vi "Read TSP Link Synchronization Line Data.vi"(8 "error in (no error)":errorcluster, 9 "TSP Link Line (1)":i32=1, 10 "Data Type (0: Bit)":i32(ring) items=["Bit", "Port"], 11 "VISA resource name":refnum<visa-resource-name>) -> (0 "error out":errorcluster, 1 "Port":i32, 2 "Bit":i32, 3 "VISA resource name out":refnum<visa-resource-name>)   [LabVIEW 2017, in "Keithley 2600 Series.lvlib"]
doc: "Returns the TSP-Link synchronization line data.\n\n<b>Note:</b>\nThis VI is not available on models 2604B, 2614B, 2634B."
uses:
  <instrlib>/Keithley 2600 Series/Keithley 2600 Series.lvlib
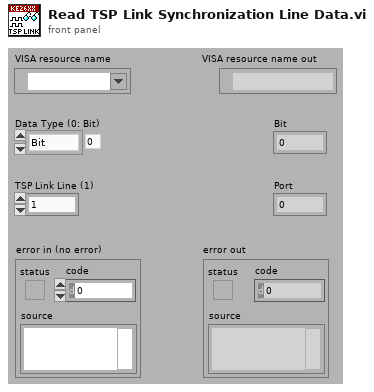
[diagram p1: front panel]
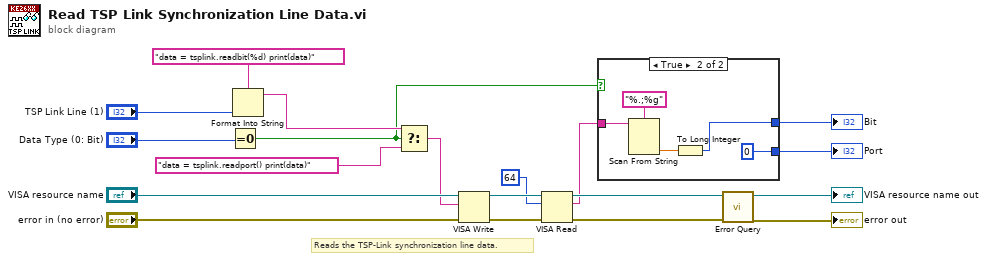
[diagram p0: block diagram]
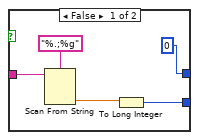
[diagram p2: hidden frame]
diagram:
  # "Reads the TSP-Link synchronization line data."
  n1 = Equal To 0?(x="Data Type (0: Bit)") -> (x = 0?=w5:bool)
  n2 = Format Into String(format string="data = tsplink.readbit(%d) print(data)", "TSP Link Line (1)") -> (resulting string=w12:string)  [unwired: 2 in, 1 out]
  n3 = Select(t=w12, s=w5, f="data = tsplink.readport() print(data)") -> (s? t:f=w1:string)
  n4 = VISA Write(VISA resource name="VISA resource name", write buffer=w1, error in (no error)="error in (no error)") -> (VISA resource name out=w10:refnum<visa-resource-name>, error out=w9:errorcluster)  [unwired: 1 out]
  n5 = VISA Read(VISA resource name=w10, byte count=u32 64, error in (no error)=w9) -> (VISA resource name out=w8:refnum<visa-resource-name>, read buffer=w4:string, error out=w7:errorcluster)  [unwired: 1 out]
  n6 = case shown="True" w5 {
    tunnel: w4 -> [w22 w28]
    tunnel: [0 w26] -> w3
    tunnel: [w21 0] -> w2
    frame False {
      n7 = Scan From String(format string="%.;%g", input string=w22) -> (output 1=w23:dbl)  [unwired: 3 in, 3 out]
      n8 = To Long Integer(number=w23) -> (32bit integer=w21:i32)
    }
    frame True {
      n9 = Scan From String(format string="%.;%g", input string=w28) -> (output 1=w27:dbl)  [unwired: 3 in, 3 out]
      n10 = To Long Integer(number=w27) -> (32bit integer=w26:i32)
    }
  }
  "Bit" <- w3
  "Port" <- w2
  n11 = call <instrlib>:"Error Query.vi"("error in (no error)"=w7, "VISA resource name"=w8) -> ("error out"=→"error out":errorcluster, "VISA resource name out"=→"VISA resource name out":refnum<visa-resource-name>)  [unwired: 6 in, 2 out]
